vi "Write Elevator Position.vi"(8 "error in (no error)":errorcluster, 10 "Elevator Position":T1 scale=1.0..4.0, 11 "Abstract Sensor Interface in":refnum<class "Abstract Sensor Interface.lvclass">) -> (0 "error out":errorcluster, 3 "Abstract Sensor Interface out":refnum<class "Abstract Sensor Interface.lvclass">)   [LabVIEW 2019, in "Abstract Sensor Interface Actor.lvlib" / "Abstract Sensor Interface.lvclass"]
uses:
  Abstract Sensor Interface.lvclass
  Sensor Interface Actor/Sensor Interface Actor/Elevator Position.ctl
  Sensor Interface Actor/Sensor Interface Actor/Sensor Interface.lvclass
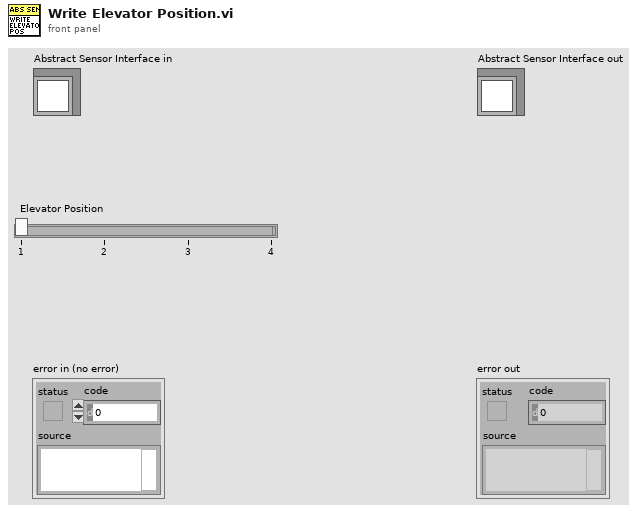
[diagram p1: front panel]
types:
  T1 = typedef "Sensor Interface Actor.lvlib/Sensor Interface.lvclass/Elevator Position.ctl" = u8
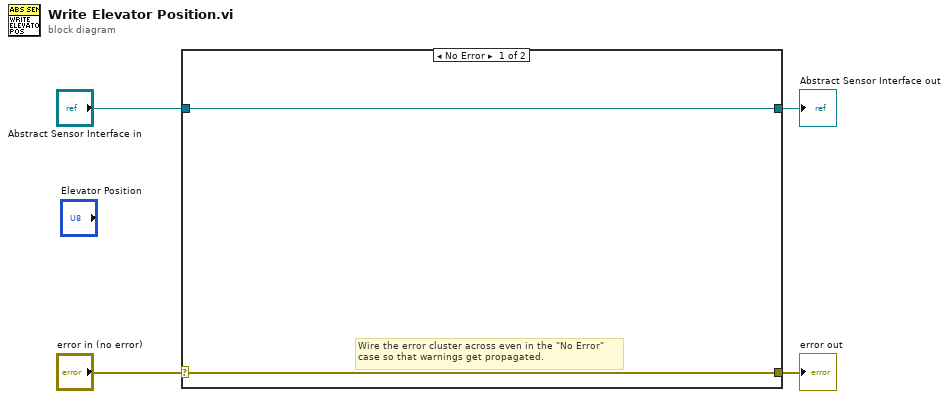
[diagram p0: block diagram]
diagram:
  n1 = case shown="No Error" "error in (no error)" {
    selector: "error in (no error)" -> [w5 w8]
    tunnel: [w5 w8] -> w3
    tunnel: [w6 w7] -> w1
    tunnel: "Abstract Sensor Interface in" -> [w6 w7]
    frame No Error {
      # "Wire the error cluster across even in the \"No Error\"\ncase so that warnings get propagated."
    }
    frame Error {
    }
  }
  "error out" <- w3
  "Abstract Sensor Interface out" <- w1
